vi "AlazarGetSystemHandle.vi"(2 "error in (no error)":errorcluster, 3 "System ID":u32) -> (0 "error out":errorcluster, 1 "Handle":u64)   [LabVIEW 2009]
doc: "Return the handle of the master board in the specified board system."
uses:
  ATSApi.dll
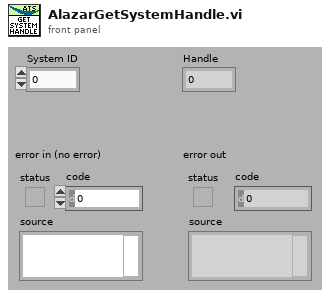
[diagram p1: front panel]
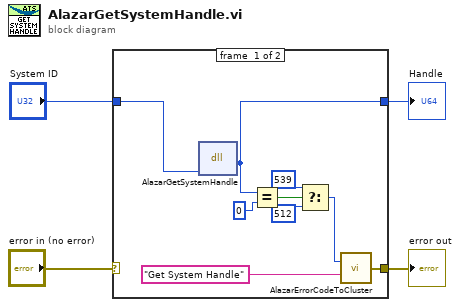
[diagram p0: block diagram]
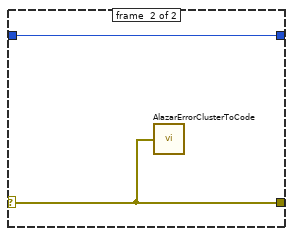
[diagram p2: hidden frame]
diagram:
  n1 = case shown="No Error" "error in (no error)" {
    selector: "error in (no error)" -> [_ w15]
    tunnel: [w11 w15] -> w3
    tunnel: "System ID" -> [w13 w14]
    tunnel: [w5 w14] -> w1
    frame #0 {
      n2 = dll-call lib="ATSApi.dll" fn="AlazarGetSystemHandle"("systemId"=w13) -> ("return type"=w5:u64)  [unwired: 4 in, 2 out]
      n3 = Equal?(x=w5, y=u64 0) -> (x = y?=w9:bool)
      n4 = Select(t=u32 539, s=w9, f=u32 512) -> (s? t:f=w6:u32)
      n5 = call "AlazarErrorCodeToCluster.vi"("Message"="Get System Handle", "Error Code"=w6) -> ("error out"=w11:errorcluster)
    }
    frame #1 {
      n6 = call "AlazarErrorClusterToCode.vi"("error in (no error)"=w15) -> ()  [unwired: 1 out]
    }
  }
  "Handle" <- w1
  "error out" <- w3
